vi "Element Type.vi"(11 "LoggingControl in":refnum<class "LoggingControl.lvclass">) -> (2 "Element Type":string)   [LabVIEW 2020, in "VolatusGUIElements.lvlib" / "LoggingControl.lvclass"]
uses:
  LoggingControl.lvclass
  LoggingControl.lvclass/LoggingControl.ctl
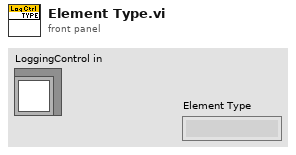
[diagram p1: front panel]
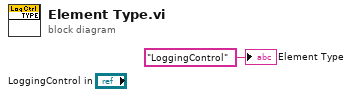
[diagram p0: block diagram]
diagram:
  "Element Type" <- "LoggingControl" ("Element Type")
